vi "Valid Response Configuration.vi"(8 "error in (no error)":errorcluster, 11 "Return Request in":T1) -> (0 "error out":errorcluster)   [LabVIEW 2017, in "SSH.lvlib"]
doc: "Sets an error if the response configuration is invalid (prevents a hang as an invalid response configuration will cause the application to go into an endless loop)"
uses:
  SSH.lvlib
  Return Request Configuration.ctl
  Response Configuration.ctl
  <vilib>/Utility/error.llb/Error Cluster From Error Code.vi
  <vilib>/ErrorRing/Error Ring.xnode
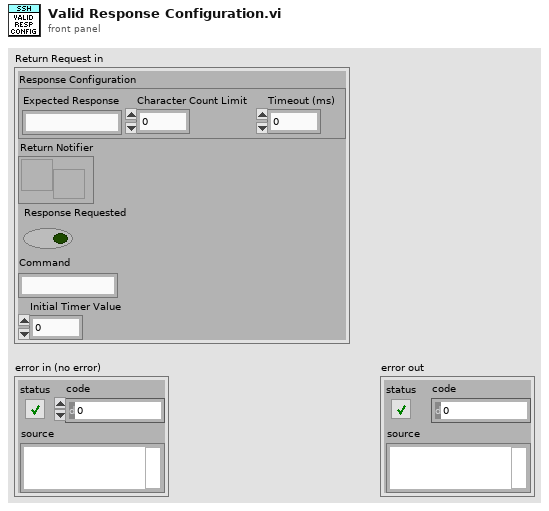
[diagram p1: front panel]
types:
  T1 = typedef "SSH.lvlib/Return Request Configuration.ctl" = cluster{"Response Configuration":T2, "Return Notifier":refnum<notifier>, "Response Requested":bool, "Command":string, "Initial Timer Value":u32}
  T2 = typedef "SSH.lvlib/Response Configuration.ctl" = cluster{"Expected Response":string, "Character Count Limit":i32, "Timeout (ms)":u32}
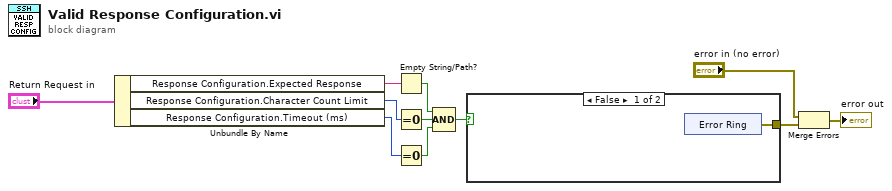
[diagram p0: block diagram]
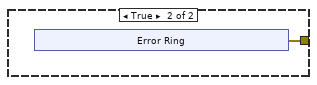
[diagram p2: hidden frame]
diagram:
  n1 = Unbundle By Name("Return Request in") -> ("Response Configuration.Expected Response"=w8:string, "Response Configuration.Character Count Limit"=w10:i32, "Response Configuration.Timeout (ms)"=w9:u32)
  n2 = Empty String/Path?(string/path=w8) -> (empty?=w7:bool)
  n3 = Equal To 0?(x=w10) -> (x = 0?=w6:bool)
  n4 = Equal To 0?(x=w9) -> (x = 0?=w5:bool)
  n5 = Compound Arithmetic op=AND(w7, w6, w5) -> (w4:bool)
  n6 = case shown="False" w4 {
    tunnel: [w12 w14] -> w2
    frame False {
      n7 = xnode "Error Ring"() -> ("error out"=w12:errorcluster)
    }
    frame True {
      n8 = xnode "Error Ring"() -> ("error out"=w14:errorcluster)
    }
  }
  n9 = Merge Errors("error in (no error)", w2) -> (→"error out":errorcluster)
